vi "PID DAQ.vi"(8 "error in":errorcluster, 10 "TDMS in":refnum<class "TDMS.lvclass">, 11 "PIDs":refnum<class "PID.lvclass">[](array[class])) -> (0 "error out":errorcluster, 2 "TDMS out":refnum<class "TDMS.lvclass">, 3 "PIDs":refnum<class "PID.lvclass">[](array[class]))   [LabVIEW 2011]
uses:
  Modules/File/TDMS/TDMS.lvclass
  Modules/Hardware/PID/PID.lvclass
  Functional Global Data/Device Params Global.ctl
  Functional Global Data/Run Data.ctl
  <vilib>/Platform/TimedLoop/XDataNode/timing_clust.ctl
  <vilib>/Platform/TimedLoop/XDataNode/nitl_modes.ctl
  <vilib>/Platform/TimedLoop/XDataNode/wakeup.ctl
  Controls/User Interface Action.ctl
  <vilib>/Platform/TimedLoop/XDataNode/XDataNode.xnode
  <vilib>/Platform/TimedLoop/XDataNode/XDNodeRunTimeDep.lvlib
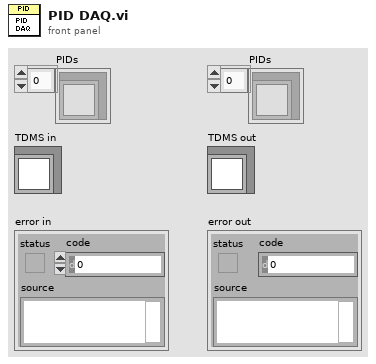
[diagram p1: front panel]
types:
  T1 = typedef "Device Params Global.ctl" = enum16{"Initialize", "Get Device Settings", "Get Device Connections", "Set Device Settings", "Set Device Connections", "Get All Device Properties"}
  T2 = typedef "Run Data.ctl" = enum16{"Initialize", "Add Sample Channel", "Set Run", "Get Number of Runs", "Set Run Params", "Get Spectrum", "Get Run Params", "Get Sample Params", "Get History", "Get Averaged History", "Get Run Param Names", "Set Run Param Names", "Get Sample Param Names", "Set Sample Param Names", "Get MFC Flow Rate Challenge Profile", "Get History Average"}
  T3 = typedef "User Interface Action.ctl" = enum16{"Initialize", "Data Acquisition Disable", "Data View Disable", "Sample Set", "Sample Set 2D Data", "Sample Set x0 & dx", "Sample Add", "Sample Set Cursor", "Sample Set Offset & Multiplier", "Sample Set Axis Labels", "Sample Parameters Disabled", "Sample Parameters Update", "Run Update", "Run Set Offset & Multiplier", "Run Set Axis Labels", "Run Set Cursor", "Run Set Disabled", "Run Parameters Update", "Run Parameters Disabled", "Run Number Set", "Run Number Set Range", "Run Number Set Disabled", "Sample Number Set", "Sample Number Set Range", "Notes Set Value", "Update Plot", "Set Plot Parameters", "Update Concentration Plot", "Time Set", "Clear DAQ Display", "Clear Analysis Display", "Status Bar Set", "Progress Bar Set", "Display Mode Set", "Experiment Type Set", "Analysis Plot Average Set", "Stop"}
  T4 = typedef "XDNodeRunTimeDep.lvlib/timing_clust.ctl" = cluster{"Expected End [f-1]":u64, "Actual End [f-1]":u64, "Finished Late? [f-1]":bool, "Expected End [i-1]":u64, "Actual End [i-1]":u64, "Finished Late? [i-1]":bool, "Expected Start [i]":u64, "Actual Start [i]":u64, "Expected Start [f]":u64, "Actual Start [f]":u64, "Source Name":string, "Structure Name":string, "Period":i64, "Deadline":i64, "Offset":i64, "Start":i64, "Priority":i32, "Timeout":i32, "Mode":T5, "Wakeup Reason":T6, "Error":errorcluster, "Source Type":string, "Secondary Source Type":string, "Global End Time":u64, "Global Start Time":u64, "Frame Duration":u64, "Iteration Duration":u64, "Assigned CPU":i32, "I/O Scan Engine Mode":u32}
  T5 = typedef "XDNodeRunTimeDep.lvlib/nitl_modes.ctl" = enum32{"No Change", "Process missed periods, maintain original phase", "Discard missed periods, maintain original phase", "Process missed periods, ignore original phase", "Discard missed periods, ignore original phase"}
  T6 = typedef "XDNodeRunTimeDep.lvlib/wakeup.ctl" = enum32{"Normal", "Aborted", "Asynchronous wakeup", "Timing source error", "Timed loop error", "Timeout"}
  T7 = typedef "Device Connections.ctl" = cluster{"Detector":cluster{"Detector Type":T8, "Connection":bool, "B-M PID":T9, "INL PID Connections":T10}, "Power Supply":cluster{"Type":enum16{"Stanford Research PS350", "Keithley 2400"}, "Connection":bool, "VISA resource name":refnum<visa-resource-name>}, "Mass Flow Controller":cluster{"Type":enum16{"Aalborg GFC17"}, "Connection":bool, "Aalborg GFC17":T12}, "Valve Controller":cluster{"Type":T13, "Connection":bool, "SMC - INL":cluster{"VISA resource name":refnum<visa-resource-name>}}, "Multimeter":cluster{"Multimeter Type":T14, "Connection":bool, "VISA resource name":refnum<visa-resource-name>}, "Vapour Generator":cluster{"Type":T15, "Connection":bool, "Owlstone Gen-SYS":T16}}
  T8 = typedef "Detector Type.ctl" = enum16{"INL PID", "Baseline-Mocon piD-TECH plus"}
  T9 = typedef "Baseline Mocon piD-Tech plus.lvclass/Connections.ctl" = cluster{"AI DAQmx channel":tag}
  T10 = typedef "INL PID Connections.ctl" = cluster{"PIDs":u8, "Integrator DAQ Channels 1":T11, "Integrator DAQ Channels 2":T11}
  T11 = typedef "INL PID.lvclass/Integrator DAQmx Channels.ctl" = cluster{"V0":tag, "S1":tag, "S2":tag}
  T12 = typedef "Aalborg GFC17.lvclass/Aalborg GFC17 Connections.ctl" = cluster{"flow rate setpoint channel":tag, "flow rate reading channel":tag, "valve channel":tag}
  T13 = typedef "Valve Type.ctl" = enum16{"SMC - INL"}
  T14 = typedef "Multimeter Type.ctl" = enum16{"Agilent 3458A"}
  T15 = typedef "Vapour Generator Type.ctl" = enum16{"Owlstone GEN-SYS"}
  T16 = typedef "Owlstone GEN-SYS.lvclass/GEN-SYS Connections.ctl" = cluster{"GEN-SYS VISA resource name":refnum<visa-resource-name>, "OVG-4":cluster{"Flow Address":u8, "Temp Address":u8}, "OHG-4":cluster{"Flow Address":u8, "Easydew VISA resource name":refnum<visa-resource-name>}}
  T17 = typedef "Device Settings.ctl" = cluster{"PID":cluster{"B-M PID":T18, "INL PID":T19}, "Power Supply":cluster{"Source Value":dbl, "Source Value Units":T20, "Source Mode":T21, "Limits":T22, "Output":bool}, "Mass Flow Controller":cluster{"MFC Flow Rate":dbl, "MFC Valve Status":T25}, "Valve Controller":cluster{"Valve Assembly":T26}, "Multimeter":cluster{"Agilent 3458A":cluster{"Measurement Configuration":T28, "Measurement Integration":T29}}, "Vapour Generator":cluster{"Owlstone Permeation Tube":T30, "Owlstone GEN-SYS Setpoints":T32}}
  T18 = typedef "Baseline Mocon piD-Tech plus.lvclass/Settings.ctl" = cluster{"Detector Sampling Frequency":dbl}
  T19 = typedef "INL PID.lvclass/Settings.ctl" = cluster{"Sampling Frequency":dbl, "Integration Time":dbl, "Integration Periods":u8, "Grid Voltage":dbl}
  T20 = typedef "Power Supply.lvclass/Source Units.ctl" = enum16{"volts", "millivolts", "microvolts", "amps", "milliamps", "microamps", "nanoamps"}
  T21 = typedef "Power Supply.lvclass/Source Mode.ctl" = enum16{"Volts", "Current"}
  T22 = typedef "Power Supply.lvclass/Protection Limits.ctl" = cluster{"Voltage Limit":dbl, "Voltage Limit Units":T23, "Current Limit":dbl, "Current Limit Units":T24, "Voltage Trip/Cmpl":dbl, "Voltage Trip/Cmpl Units":T23, "Current Trip/Cmpl":dbl, "Current Trip/Cmpl Units":T24}
  T23 = typedef "Power Supply.lvclass/Voltage Units.ctl" = enum16{"volts", "millivolts", "microvolts"}
  T24 = typedef "Power Supply.lvclass/Current Units.ctl" = enum16{"amps", "milliamps", "microamps", "nanoamps"}
  T25 = typedef "Mass Flow Controller.lvclass/Valve Status.ctl" = enum16{"Open", "Closed"}
  T26 = typedef "Valve Controller.lvclass/Valve Assembly.ctl" = cluster{"Valve 1":T27, "Valve 2":T27, "Valve 3":T27, "Valve 4":T27, "Valve 5":T27}
  T27 = typedef "Valve Controller.lvclass/Status.ctl" = u16
  T28 = typedef "Agilent 3458A.lvclass/Measurement Configuration.ctl" = cluster{"Function":enum16{"DC Voltage", "AC Voltage", "AC + DC Voltage", "DC Current", "AC Current", "AC + DC Current", "2-Wire Resistance", "4-Wire Resistance", "Frequency", "Period", "Direct Sampling DC", "Direct Sampling AC", "Sub-Sampling DC", "Sub-Sampling AC"}, " Manual Resolution":enum16{"4.5", "5.5", "6.5", "7.5", "8.5"}, "Frequency Source":enum16{"AC + DC Current", "AC + DC Voltage", "AC Current", "AC Voltage"}, "Auto Range":enum16{"OFF", "ON", "ONCE"}}
  T29 = typedef "Agilent 3458A.lvclass/Measurement Integration.ctl" = cluster{"Power Line Cycles":dbl}
  T30 = typedef "Owlstone GEN-SYS.lvclass/Permeation Tube.ctl" = cluster{"Tube":T31, "Molecular Weight":dbl, "Calibration Temperature\n(Celcius)":i32, "Permeation Rate \n(ng/min)":i32}
  T31 = typedef "Owlstone GEN-SYS.lvclass/Permeation Tube Gas.ctl" = enum16{"Isobutylene 27 Nov 2012", "Ammonia 29 Sep 2012", "DMMP Tube A 3 July 2014", "DMMP Tube B 3 July 2014"}
  T32 = typedef "Owlstone GEN-SYS.lvclass/Gen-Sys Setpoints.ctl" = cluster{"OVG-4":cluster{"Oven Temperature":i32, "Sample Flow Rate":i32, "Split Flow Status":u16, "Split Flow Rate":i32}, "OHG-4":cluster{"Wet Air Flow":i32}}
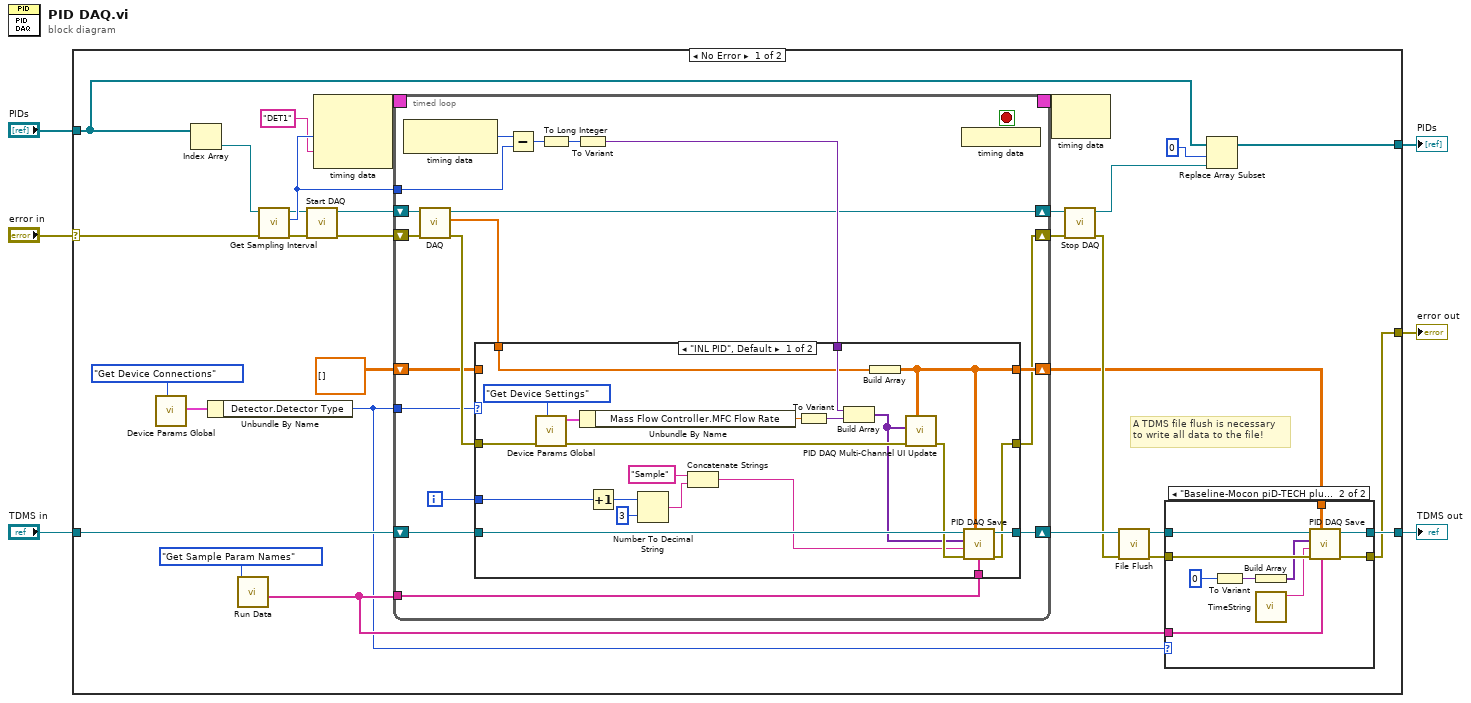
[diagram p0: block diagram]
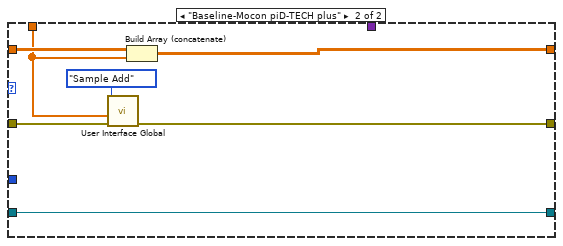
[diagram p3: hidden frame]
diagram:
  n1 = case shown="No Error" "error in" {
    selector: "error in" -> [w24 w105]
    tunnel: [w14 w105] -> w6
    tunnel: [w17 w104] -> w5
    tunnel: "TDMS in" -> [w27 w104]
    tunnel: "PIDs" -> [w11 w103]
    tunnel: [w9 w103] -> w1
    frame No Error {
      # "A TDMS file flush is necessary\nto write all data to the file!"
      n2 = call "Device Params Global.vi"("action"=Device_Params_Global."Get Device Connections") -> ("Device Connections OUT"=w21:T7)  [unwired: 8 in, 2 out]
      n3 = Index Array(array=w11) -> (element=w12:refnum<class "PID.lvclass">)  [unwired: 1 in]
      n4 = Unbundle By Name(w21) -> ("Detector.Detector Type"=w13:T8)
      n5 = call "Run Data.vi"("action"=Run_Data."Get Sample Param Names" ("Action")) -> ("Param Names OUT"=w15:string[])  [unwired: 7 in, 3 out]
      n6 = call-dynamic "Get Sampling Interval.vi"("error in (no error)"=w24, "PID in"=w12) -> ("error out"=w32:errorcluster, "Sampling Interval"=w34:u32, "PID out"=w33:refnum<class "PID.lvclass">)  [unwired: 7 in]
      n7 = call-dynamic "Start DAQ.vi"("error in (no error)"=w32, "Detector in"=w33) -> ("error out"=w7:errorcluster, "Detector out"=w29:refnum<class "PID.lvclass">)  [unwired: 8 in]
      n8 = node-c288(w34, "DET1" ("Name")) -> (w36:T4)  [unwired: 1 in]
      n9 = timed-loop {
        timing: w36 -> [_]
        timing-out: [_] -> w35
        shift-right: [w58] -> w30
        shift-left: w29 -> [w65]
        shift-right: [w51] -> w28
        shift-left: w27 -> [w52]
        shift-right: [w49] -> w31
        shift-left: w7 -> [w64]
        tunnel: w34 -> [w60]
        tunnel: w15 -> [w50]
        tunnel: w13 -> [w55]
        shift-right: [w53] -> w18
        shift-left: dbl[][] [] ("data") -> [w54]
        i -> [w66]
        stop <- _ stop-if-true
        n10 = node-c288() -> (w61:i64)  [unwired: 1 in]
        n11 = call-dynamic "DAQ.vi"("error in"=w64, "Detector in"=w65) -> ("error out"=w56:errorcluster, "data"=w57:dbl[], "Detector out"=w58:refnum<class "PID.lvclass">)  [unwired: 7 in]
        n12 = Subtract(x=w61, y=w60) -> (x-y=w59:i64)
        n13 = To Long Integer(number=w59) -> (32bit integer=w62:i32)
        n14 = To Variant(anything=w62) -> (Variant=w63:variant)
        n15 = case shown="\"INL PID\", Default" w55 {
          tunnel: w66 -> [w87 _]
          tunnel: w63 -> [w83 _]
          tunnel: w57 -> [w68 w88]
          tunnel: w56 -> [w76 w91]
          tunnel: w54 -> [_ w94]
          tunnel: [w71 w90] -> w49
          tunnel: [w67 w93] -> w53
          tunnel: w52 -> [w75 w89]
          tunnel: [w74 w89] -> w51
          tunnel: w50 -> [w73 _]
          frame "INL PID", Default {
            n16 = call "Device Params Global.vi"("action"=Device_Params_Global."Get Device Settings", "error in"=w76) -> ("error out"=w79:errorcluster, "Device Settings OUT"=w85:T17)  [unwired: 7 in, 1 out]
            n17 = Unbundle By Name(w85) -> ("Mass Flow Controller.MFC Flow Rate"=w80:dbl)
            n18 = Increment(x=w87) -> (x+1=w78:i32)
            n19 = Number To Decimal String(number=w78, width (-)=i16 3) -> (decimal integer string=w81:string)
            n20 = Concatenate Strings("Sample" ("string"), w81) -> (w69:string)
            n21 = To Variant(anything=w80) -> (Variant=w84:variant)
            n22 = Build Array(w83, w84) -> (w70:variant[])
            n23 = Build Array(w68) -> (w67:dbl[][])
            n24 = call "PID DAQ Multi-Channel UI Update.vi"("Sample Data"=w67, "error in"=w79, "Sample Parameter"=w70) -> ("error out"=w72:errorcluster)  [unwired: 8 in]
            n25 = call "PID DAQ Save.vi"("Sample Parameter Names"=w73, "Sample Data"=w67, "error in"=w72, "Sample Name"=w69, "Sample Parameters"=w70, "TDMS in"=w75) -> ("error out"=w71:errorcluster, "TDMS out"=w74:refnum<class "TDMS.lvclass">)  [unwired: 4 in]
          }
          frame "Baseline-Mocon piD-TECH plus" {
            n26 = call "User Interface Global.vi"("error in"=w91, "data1"=w88, "action"=User_Interface_Action."Sample Add") -> ("error out"=w90:errorcluster)  [unwired: 8 in]
            n27 = Build Array (concatenate)(w94, w88) -> (w93:dbl[][])
          }
        }
        n28 = node-c288() -> ()  [unwired: 1 out]
      }
      n29 = node-c288(w35) -> ()  [unwired: 1 out]
      n30 = call-dynamic "Stop DAQ.vi"("error in (no error)"=w31, "Detector in"=w30) -> ("error out"=w23:errorcluster, "Detector out"=w10:refnum<class "PID.lvclass">)  [unwired: 8 in]
      n31 = call-dynamic "File Flush.vi"("error in"=w23, "TDMS in"=w28) -> ("error out"=w16:errorcluster, "TDMS out"=w19:refnum<class "TDMS.lvclass">)  [unwired: 8 in]
      n32 = case shown="\"Baseline-Mocon piD-TECH plus\"" w13 {
        tunnel: w19 -> [w38 w46]
        tunnel: w18 -> [_ w45]
        tunnel: [w38 w44] -> w17
        tunnel: w16 -> [w37 w43]
        tunnel: w15 -> [_ w41]
        tunnel: [w37 w39] -> w14
        frame "INL PID", Default {
        }
        frame "Baseline-Mocon piD-TECH plus" {
          n33 = To Variant(anything=0) -> (Variant=w48:variant)
          n34 = Build Array(w48) -> (w40:variant[])
          n35 = call "TimeString.vi"() -> ("String"=w42:string)  [unwired: 11 in]
          n36 = call "PID DAQ Save.vi"("Sample Parameter Names"=w41, "Sample Data"=w45, "error in"=w43, "Sample Name"=w42, "Sample Parameters"=w40, "TDMS in"=w46) -> ("error out"=w39:errorcluster, "TDMS out"=w44:refnum<class "TDMS.lvclass">)  [unwired: 4 in]
        }
      }
      n37 = Replace Array Subset(array=w11, new element=w10, index=0) -> (w9:refnum<class "PID.lvclass">[])
    }
    frame Error {
    }
  }
  "error out" <- w6
  "TDMS out" <- w5
  "PIDs" <- w1
